vi "ClusterEscala.vi"() -> ()   [LabVIEW 2020]
panel:
  out "Cluster 2":T1 {"Tank" scale=0.0..10.0; "Gauge" scale=0.0..10.0; "Thermometer" scale=0.0..100.0}
  in  "Cluster":T2
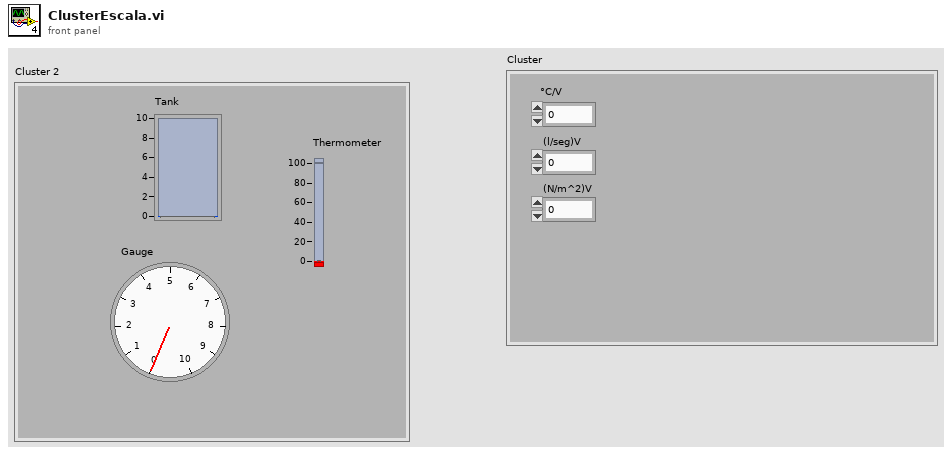
[diagram p1: front panel]
types:
  T1 = cluster{"Thermometer":dbl, "Gauge":dbl, "Tank":dbl}
  T2 = cluster{"°C/V":dbl, "(l/seg)V":dbl, "(N/m^2)V":dbl}
  T3 = cluster{"(l/seg)V":i32, "(N/m^2)V":i32, "°C/V":i32}
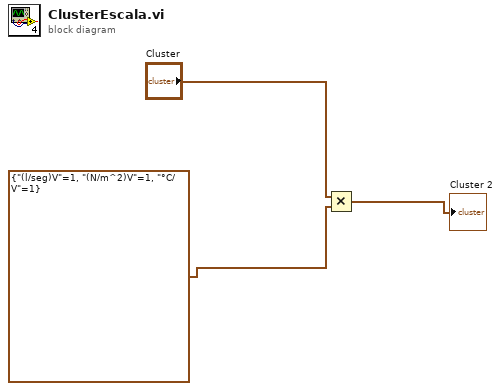
[diagram p0: block diagram]
diagram:
  n1 = Multiply(x="Cluster", y=T3 {"(l/seg)V"=1, "(N/m^2)V"=1, "°C/V"=1}) -> (x*y=→"Cluster 2":cluster{dbl, dbl, dbl})
